vi "Authorization Encode XML.vi"(8 "error in (no error)":errorcluster, 10 "Volume Serial Number":string, 11 "Decoded XML String":string) -> (0 "error out":errorcluster, 3 "Encoded XML String":string)   [LabVIEW 2011]
uses:
  <vilib>/xml/Load XML String.vi
  <vilib>/xml/Close Reference(Node).vi
  <vilib>/xml/NI_XML.lvlib
  LabVIEW 2011/resource/objmgr/DOMUserDefRef.rc
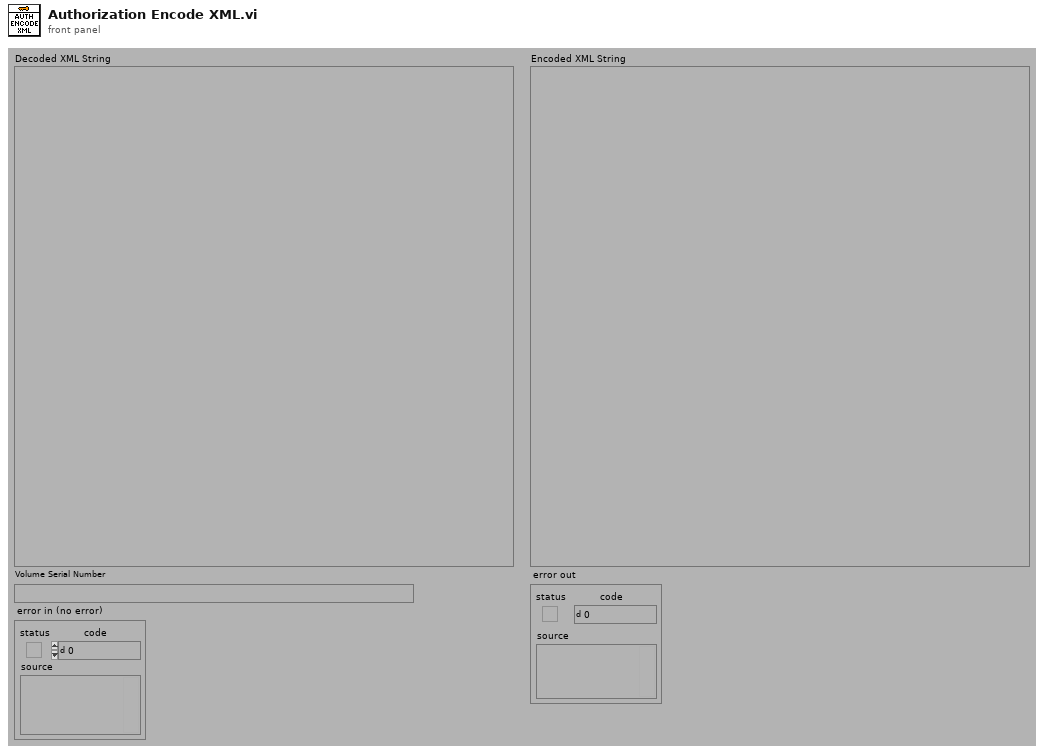
[diagram p1: front panel]
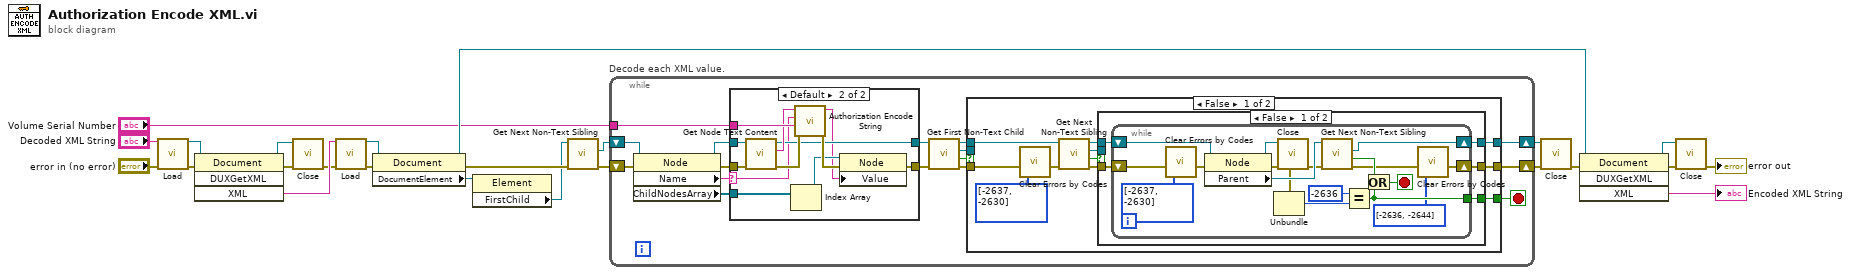
[diagram p0: block diagram]
diagram:
  n1 = call-poly <vilib>:"Load.vi"("XML string"="Decoded XML String", "error in (no error)"="error in (no error)") -> ("DOM document out"=w23:refnum<k20>, "error out"=w22:errorcluster)  [unwired: 11 in, 1 out]
  n2 = invoke class="Document" method="DUXGetXML"(reference=w23, error in=w22) -> (reference out=w20:refnum<k20>, error out=w21:errorcluster, "XML"=w19:string)  [unwired: 2 in, 1 out]
  n3 = call-poly <vilib>:"Close.vi"("error in (no error)"=w21, "node"=w20) -> ("error out"=w18:errorcluster)  [unwired: 7 in]
  n4 = call-poly <vilib>:"Load.vi"("XML string"=w19, "error in (no error)"=w18) -> ("DOM document out"=w17:refnum<k20>, "error out"=w16:errorcluster)  [unwired: 11 in, 1 out]
  n5 = property on="Property Node" class="Document"(reference=w17, error in=w16) -> (reference out=w8:refnum<k20>, error out=w14:errorcluster, "DocumentElement"=w15:refnum<k20>)
  n6 = property on="Property Node" class="Element"(reference=w15) -> ("FirstChild"=w13:refnum<k20>)  [unwired: 1 in, 2 out]
  n7 = call <vilib>:"Get Next Non-Text Sibling.vi"("error in (no error)"=w14, "node in"=w13) -> ("error out"=w12:errorcluster, "sibling node"=w11:refnum<k20>)  [unwired: 6 in, 2 out]
  n8 = while "Decode each XML value." {
    shift-right: [w40] -> w10
    shift-left: w12 -> [w38]
    shift-right: [w39] -> w9
    shift-left: w11 -> [w36]
    tunnel: "Volume Serial Number" -> [w32]
    stop <- w34 stop-if-true
    n9 = property class="Node"(reference=w36, error in=w38) -> (reference out=w35:refnum<k20>, error out=w37:errorcluster, "Name"=w25:string, "ChildNodesArray"=w33:refnum<k20>[])
    n10 = case shown="Default" w25 {
      selector: w25 -> [_ w44]
      tunnel: w37 -> [w42 w54]
      tunnel: w35 -> [w41 w53]
      tunnel: w33 -> [_ w52]
      tunnel: w32 -> [_ w51]
      tunnel: [w41 w47] -> w27
      tunnel: [w42 w45] -> w26
      frame "Feature" {
      }
      frame Default {
        n11 = call <vilib>:"Get Node Text Content.vi"("error in (no error)"=w54, "node in"=w53) -> ("error out"=w49:errorcluster, "node text"=w48:string, "node out"=w47:refnum<k20>)  [unwired: 7 in]
        n12 = Index Array(array=w52) -> (element=w46:refnum<k20>)  [unwired: 1 in]
        n13 = call "Authorization Encode String.vi"("error in (no error)"=w49, "Volume Serial Number"=w51, "Property Name"=w44, "Decoded String"=w48) -> ("error out"=w50:errorcluster, "Encoded String"=w43:string)  [unwired: 6 in]
        n14 = property class="Node"(reference=w46, error in=w50, "Value"=w43) -> (error out=w45:errorcluster)  [unwired: 1 out]
      }
    }
    n15 = call <vilib>:"Get First Non-Text Child.vi"("error in (no error)"=w26, "node in"=w27) -> ("error out"=w30:errorcluster, "found child node?"=w31:bool, "child node"=w29:refnum<k20>, "node out"=w28:refnum<k20>)  [unwired: 6 in]
    n16 = case shown="False" w31 {
      tunnel: w30 -> [w57 w90]
      tunnel: w29 -> [_ w91]
      tunnel: w28 -> [w65 _]
      tunnel: [w60 w91] -> w39
      tunnel: [w61 w90] -> w40
      tunnel: [w58 _] -> w34
      frame False {
        n17 = call "Clear Errors by Codes.vi"("Error Codes\nto Clear (Empty)"=i32[] [-2637, -2630], "error in (no error)"=w57) -> ("error out"=w56:errorcluster)  [unwired: 5 in]
        n18 = call <vilib>:"Get Next Non-Text Sibling.vi"("error in (no error)"=w56, "node in"=w65) -> ("error out"=w64:errorcluster, "found sibling node?"=w63:bool, "sibling node"=w62:refnum<k20>, "node out"=w59:refnum<k20>)  [unwired: 6 in]
        n19 = case shown="False" w63 {
          tunnel: w64 -> [w66 w89]
          tunnel: w62 -> [_ w88]
          tunnel: [w68 w89] -> w61
          tunnel: [w69 w88] -> w60
          tunnel: w59 -> [w70 _]
          tunnel: [w67 _] -> w58
          frame False {
            n20 = while {
              shift-right: [w84] -> w69
              shift-left: w70 -> [w87]
              shift-right: [w73] -> w68
              shift-left: w66 -> [w78]
              tunnel: [w76] -> w67
              stop <- w82 stop-if-true
              n21 = call "Clear Errors by Codes.vi"("Error Codes\nto Clear (Empty)"=i32[] [-2637, -2630], "error in (no error)"=w78) -> ("error out"=w77:errorcluster)  [unwired: 5 in]
              n22 = property class="Node"(reference=w87, error in=w77) -> (reference out=w86:refnum<k20>, error out=w71:errorcluster, "Parent"=w85:refnum<k20>)
              n23 = Unbundle(w71) -> ("code"=w80:i32)  [unwired: 2 out]
              n24 = call-poly <vilib>:"Close.vi"("error in (no error)"=w71, "node"=w86) -> ("error out"=w72:errorcluster)  [unwired: 7 in]
              n25 = call <vilib>:"Get Next Non-Text Sibling.vi"("error in (no error)"=w72, "node in"=w85) -> ("error out"=w74:errorcluster, "found sibling node?"=w83:bool, "sibling node"=w84:refnum<k20>)  [unwired: 6 in, 1 out]
              n26 = Equal?(x=-2636, y=w80) -> (x = y?=w76:bool)
              n27 = Or(x=w83, y=w76) -> (x .or. y?=w82:bool)
              n28 = call "Clear Errors by Codes.vi"("Error Codes\nto Clear (Empty)"=i32[] [-2636, -2644], "error in (no error)"=w74) -> ("error out"=w73:errorcluster)  [unwired: 5 in]
            }
          }
          frame True {
          }
        }
      }
      frame True {
      }
    }
  }
  n29 = call-poly <vilib>:"Close.vi"("error in (no error)"=w10, "node"=w9) -> ("error out"=w7:errorcluster)  [unwired: 7 in]
  n30 = invoke class="Document" method="DUXGetXML"(reference=w8, error in=w7) -> (reference out=w5:refnum<k20>, error out=w6:errorcluster, "XML"=→"Encoded XML String":string)  [unwired: 2 in, 1 out]
  n31 = call-poly <vilib>:"Close.vi"("error in (no error)"=w6, "node"=w5) -> ("error out"=→"error out":errorcluster)  [unwired: 7 in]
